vi "smsDbAvl.vi"() -> ()   [LabVIEW 2012]
uses:
  <vilib>/Platform/TimedLoop/XDataNode/timing_clust.ctl
  <vilib>/Platform/TimedLoop/XDataNode/nitl_modes.ctl
  <vilib>/Platform/TimedLoop/XDataNode/wakeup.ctl
  <vilib>/addons/database/Auxilliary.llb/DB Tools Cursor Type.ctl
  <vilib>/addons/database/Connection.llb/DB Tools Open Connec (Path).vi
  <vilib>/addons/database/Connection.llb/Conn Execute.vi
  <vilib>/addons/database/Recordset.llb/Rec Get Recordset Properties (R).vi
  <vilib>/addons/database/Recordset.llb/Rec Fetch String Data (R).vi
  <vilib>/addons/database/Recordset.llb/Rec Destroy - Connection.vi
  <vilib>/platform/TimedLoop/XDataNode/XDataNode.xnode
  <vilib>/addons/database/NI_Database_API.lvlib
  <vilib>/Platform/TimedLoop/XDataNode/XDNodeRunTimeDep.lvlib
panel:
  in  "stop":bool
  in  "SMS":bool
  in  "VISA resource name":refnum<visa-resource-name>="COM17"
  in  "Control":T1(tab)
  in  "Password":string
  in  "APN":T2
  in  "IP/Port":T3
  in  "DNS":T4
  in  "GPRS":bool
  in  "Intervalo":T5
  in  "I/O":bool
  in  "POC":u16(ring) items=["POC 1", "POC 2", "POC 3", "POC 4", "POC 5", "POC 6", "POC 7", "POC 8", "POC 9", "POC 10", "POC 11", "POC 12", "POC 13", "POC 14", "POC 15", "POC 16", "POC 17", "POC 18", "POC 19", "POC 20", "POC 21", "POC 22", "POC 23", "POC 24", "POC 25", "POC 26", "POC 27", "POC 28", "POC 29", "POC 30", "POC 31", "POC 32", "POC 33", "POC 34", "POC 35", "POC 36", "POC 37", "POC 38", "POC 39", "POC 40", "POC 41", "POC 42", "POC 43", "POC 44", "POC 45", "POC 46", "POC 47", "POC 48", "POC 49", "POC 50", "POC 51", "POC 52", "POC 53", "POC 54", "POC 55", "POC 56", "POC 57", "POC 58", "POC 59", "POC 60", "POC 61", "POC 62", "POC 63", "POC 64", "POC 65", "POC 66", "POC 67", "POC 68", "POC 69", "POC 70", "POC 71", "POC 72", "POC 73", "POC 74", "POC 75", "POC 76", "POC 77", "POC 78", "POC 79", "POC 80", "POC 81", "POC 82", "POC 83", "POC 84", "POC 85", "POC 86", "POC 87", "POC 88", "POC 89", "POC 90", "POC 91", "POC 92", "POC 93", "POC 94", "POC 95", "POC 96", "POC 97", "POC 98", "POC 99", "POC 100"]
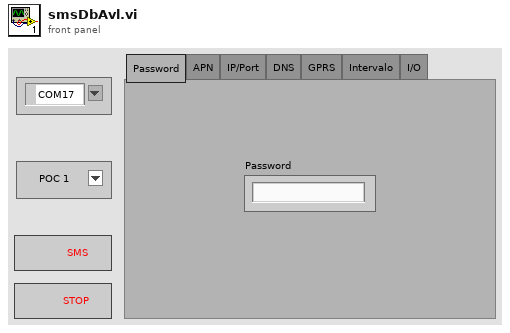
[diagram p1: front panel]
types:
  T1 = enum32{"Password", "APN", "IP/Port", "DNS", "GPRS", "Intervalo", "I/O"}
  T2 = cluster{"APN":string, "APN USER":string, "APN PASSWORD":string}
  T3 = cluster{"ip dns":bool, "IP/DNS":string, "Port":string}
  T4 = cluster{"State":bool, "DNS2":string, "DNS1":string}
  T5 = cluster{"Intervalo [Seg]":string, "Veces":string}
  T6 = typedef "NI_Database_API.lvlib/Conn ObjectReference.ctl" = refnum<k1>
  T7 = typedef "XDNodeRunTimeDep.lvlib/timing_clust.ctl" = cluster{"Expected End [f-1]":u64, "Actual End [f-1]":u64, "Finished Late? [f-1]":bool, "Expected End [i-1]":u64, "Actual End [i-1]":u64, "Finished Late? [i-1]":bool, "Expected Start [i]":u64, "Actual Start [i]":u64, "Expected Start [f]":u64, "Actual Start [f]":u64, "Source Name":string, "Structure Name":string, "Period":i64, "Deadline":i64, "Offset":i64, "Start":i64, "Priority":i32, "Timeout":i32, "Mode":T8, "Wakeup Reason":T9, "Error":errorcluster, "Source Type":string, "Secondary Source Type":string, "Global End Time":u64, "Global Start Time":u64, "Frame Duration":u64, "Iteration Duration":u64, "Assigned CPU":i32, "I/O Scan Engine Mode":u32}
  T8 = typedef "XDNodeRunTimeDep.lvlib/nitl_modes.ctl" = enum32{"No Change", "Process missed periods, maintain original phase", "Discard missed periods, maintain original phase", "Process missed periods, ignore original phase", "Discard missed periods, ignore original phase"}
  T9 = typedef "XDNodeRunTimeDep.lvlib/wakeup.ctl" = enum32{"Normal", "Aborted", "Asynchronous wakeup", "Timing source error", "Timed loop error", "Timeout"}
  T10 = enum16{"Imei", "POC", "Evento", "Lat", "Lon", "F_H_eve", "F_H_rec", "AVL_N", "AVL_pass", "Propietario", "Razon_Social", "Direccion", "Propietario_N", "Ciudad", "Marca", "Ruta", "N_Ruta", "Auditor", "Auditor_N", "Icon"}
  T11 = enum16{"POC", "Imei", "Evento", "Lat", "Lon", "F_H_eve", "F_H_rec", "AVL_N", "AVL_pass", "Propietario", "Razon_Social", "Direccion", "Propietario_N", "Ciudad", "Marca", "Ruta", "N_Ruta", "Auditor", "Auditor_N"}
  T12 = typedef "NI_Database_API.lvlib/DB Tools Cursor Type.ctl" = enum16{"forward-only", "keyset", "dynamic", "static"}
  T13 = cluster{"VISA resource name":refnum<visa-resource-name>, "Pass":string, "NUMERO":string}
  T14 = typedef "NI_Database_API.lvlib/Rec ObjectReference.ctl" = refnum<k1>
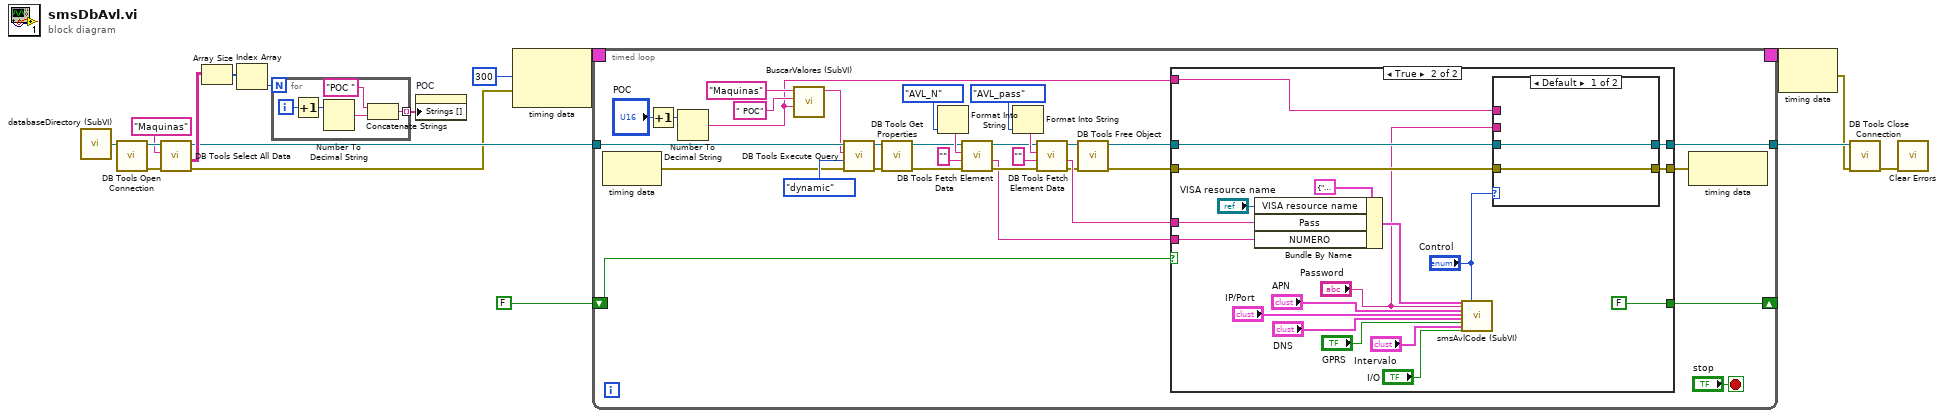
[diagram p0: block diagram]
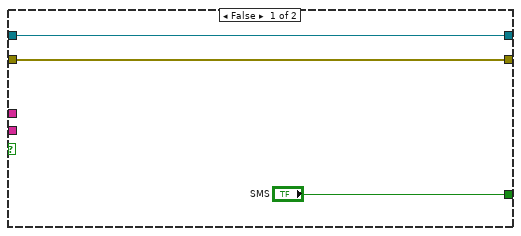
[diagram p2: hidden frame]
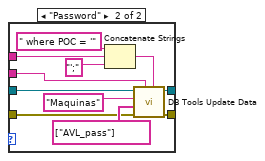
[diagram p3: hidden frame]
diagram:
  n1 = call "databaseDirectory (SubVI).vi"() -> ("Application Directory"=w3:path)  [unwired: 1 in]
  n2 = call-poly <vilib>:"DB Tools Open Connection.vi"("connection information"=w3) -> ("error out"=w15:errorcluster, "connection reference"=w14:T6)  [unwired: 7 in]
  n3 = call <vilib>:"DB Tools Select All Data.vi"("error in (no error)"=w15, "table"="Maquinas", "connection reference"=w14) -> ("error out"=w7:errorcluster, "data"=w17:string[][], "connection reference out"=w10:T6)  [unwired: 3 in]
  n4 = Array Size(array=w17) -> (size(s)=w16:i32[])
  n5 = Index Array(array=w16) -> (element=w12:i32)  [unwired: 1 in]
  n6 = for {
    N: w12 -> [_]
    tunnel: [w19] -> w11 mode=indexing
    i -> [w21]
    n7 = Increment(x=w21) -> (x+1=w22:i32)
    n8 = Number To Decimal String(number=w22) -> (decimal integer string=w20:string)  [unwired: 1 in]
    n9 = Concatenate Strings("POC " ("string"), w20) -> (w19:string)
  }
  n10 = property on="POC" class="Ring (strict)"("Strings []"=w11) -> ()  [unwired: 2 in, 2 out]
  n11 = node-c288(i64 300 ("Period"), w7) -> (w9:T7)
  n12 = timed-loop {
    timing: w9 -> [_]
    timing-out: [_] -> w8
    tunnel: [w29] -> w2
    tunnel: w10 -> [w54]
    shift-right: [w35] -> _
    shift-left: FALSE ("SMS") -> [w34]
    stop <- "stop" stop-if-true
    n13 = node-c288() -> (w36:errorcluster)  [unwired: 1 in]
    n14 = Increment(x="POC") -> (x+1=w41:u16)
    n15 = Number To Decimal String(number=w41) -> (decimal integer string=w23:string)  [unwired: 1 in]
    n16 = call "BuscarValores (SubVI).vi"("="=w23, "Columna"=" POC" ("Substring"), "Tabla"="Maquinas" ("table")) -> ("String"=w30:string)  [unwired: 8 in]
    n17 = call-poly <vilib>:"DB Tools Execute Query.vi"("error in (no error)"=w36, "cursor type"=DB_Tools_Cursor_Type."dynamic", "SQL query"=w30, "connection reference"=w54) -> ("error out"=w49:errorcluster, "recordset reference"=w50:T14)  [unwired: 4 in]
    n18 = call-poly <vilib>:"DB Tools Get Properties.vi"("error in (no error)"=w49, "recordset reference"=w50) -> ("error out"=w44:errorcluster, "recordset reference out"=w45:T14)  [unwired: 3 in, 1 out]
    n19 = Format Into String(T10."AVL_N") -> (resulting string=w46:string)  [unwired: 3 in, 1 out]
    n20 = call-poly <vilib>:"DB Tools Fetch Element Data.vi"("error in (no error)"=w44, "type"="", "column index"=w46, "recordset reference"=w45) -> ("error out"=w42:errorcluster, "data"=w37:string, "recordset reference out"=w43:T14)  [unwired: 3 in]
    n21 = Format Into String(T11."AVL_pass") -> (resulting string=w53:string)  [unwired: 3 in, 1 out]
    n22 = call-poly <vilib>:"DB Tools Fetch Element Data.vi"("error in (no error)"=w42, "type"="", "column index"=w53, "recordset reference"=w43) -> ("error out"=w26:errorcluster, "data"=w38:string, "recordset reference out"=w27:T14)  [unwired: 3 in]
    n23 = call-poly <vilib>:"DB Tools Free Object.vi"("error in (no error)"=w26, "recordset reference"=w27) -> ("error out"=w24:errorcluster, "connection reference"=w25:T6)  [unwired: 8 in]
    n24 = case shown="True" w34 {
      tunnel: w38 -> [_ w68]
      tunnel: w37 -> [_ w67]
      tunnel: ["SMS" FALSE ("SMS")] -> w35
      tunnel: w25 -> [w56 w63]
      tunnel: w24 -> [w55 w64]
      tunnel: [w56 w61] -> w29
      tunnel: [w55 w62] -> w28
      tunnel: w23 -> [_ w60]
      frame False {
      }
      frame True {
        n25 = Bundle By Name(cluster=T13 {"VISA resource name"="", "Pass"="", "NUMERO"=""} ("Iniciar"), "VISA resource name"="VISA resource name", "Pass"=w68, "NUMERO"=w67) -> (w70:T13)
        n26 = call "smsAvlCode (SubVI).vi"("Iniciar"=w70, "Password"="Password", "APN"="APN", "IP/Port"="IP/Port", "DNS"="DNS", "GPRS"="GPRS", "Intervalo"="Intervalo", "I/O"="I/O", "Comando"="Control") -> ()  [unwired: 19 in]
        n27 = case shown="Default" "Control" {
          tunnel: w64 -> [w77 w84]
          tunnel: w63 -> [w78 w83]
          tunnel: [w77 w82] -> w62
          tunnel: [w78 w81] -> w61
          tunnel: w60 -> [_ w80]
          tunnel: "Password" -> [_ w79]
          frame Default {
          }
          frame "Password" {
            n28 = Concatenate Strings(" where POC = '" ("Substring"), w80, "';") -> (w87:string)
            n29 = call <vilib>:"DB Tools Update Data.vi"("condition"=w87, "data"=w79, "error in (no error)"=w84, "columns"=string[] ["AVL_pass"], "table"="Maquinas", "connection reference"=w83) -> ("error out"=w82:errorcluster, "connection reference out"=w81:T6)  [unwired: 4 in]
          }
        }
      }
    }
    n30 = node-c288(w28) -> ()  [unwired: 1 out]
  }
  n31 = node-c288(w8) -> (w1:errorcluster)
  n32 = call <vilib>:"DB Tools Close Connection.vi"("error in (no error)"=w1, "connection reference"=w2) -> ("error out"=w4:errorcluster)  [unwired: 5 in]
  n33 = call <vilib>:"Clear Errors.vi"("error in (no error)"=w4) -> ()  [unwired: 6 in, 1 out]
